vi "Read Power No Objects.vi"(8 "error in (no error)":errorcluster, 10 "VISA Resource Name":refnum<visa-resource-name>, 11 "Cluster In":T2={"Wavelength"=0.0, "AVG"=0, "Range"=0, "Backlight"=0, "Beeper"=0, "Zero"=0, "Local Lockout"=0, "ATTN"=0, "Run/Stop"=0, "Units"=0, "Averaging Time"=0.5, "Averaging"=FALSE, "Most Recent Power"=5.5, "Filter"=1} {"AVG" items=["Slow"=1, "Medium"=2, "Fast"=3]; "Range" items=["Auto", "Lowest", "2", "3", "4", "5", "6", "7", "Highest"]; "Backlight" items=["Off", "Low", "High"]; "Beeper" items=["Off", "On"]; "Zero" items=["Off", "On"]; "Local Lockout" items=["Off", "On"]; "ATTN" items=["Off", "On"]; "Run/Stop" items=["Stop", "Run"]; "Units" items=["W"=1, "dB"=2, "dBm"=3, "REL"=4]; "Filter" items=["Orange"=1, "Green"=2, "Yellow"=3]}) -> (0 "error out":errorcluster, 1 "Current Power w/ Units":string, 2 "Current Power":dbl[unit], 3 "Cluster Out":T2={"Wavelength"=0.0, "AVG"=0, "Range"=0, "Backlight"=0, "Beeper"=0, "Zero"=0, "Local Lockout"=0, "ATTN"=0, "Run/Stop"=0, "Units"=0, "Averaging Time"=0.5, "Averaging"=FALSE, "Most Recent Power"=5.5, "Filter"=1} {"AVG" items=["Slow"=1, "Medium"=2, "Fast"=3]; "Range" items=["Auto", "Lowest", "2", "3", "4", "5", "6", "7", "Highest"]; "Backlight" items=["Off", "Low", "High"]; "Beeper" items=["Off", "On"]; "Zero" items=["Off", "On"]; "Local Lockout" items=["Off", "On"]; "ATTN" items=["Off", "On"]; "Run/Stop" items=["Stop", "Run"]; "Units" items=["W"=1, "dB"=2, "dBm"=3, "REL"=4]; "Filter" items=["Orange"=1, "Green"=2, "Yellow"=3]})   [LabVIEW 2009]
doc: "Advanced Read for Power Meter.\n\nPerforms time-based Averaging based of member data. Checks for erroneous data points due to auto-ranging. Also has formatted power output."
uses:
  Newport 1830-C/Public/Filters.ctl
  Newport 1830-C/Newport 1830-C.lvlib
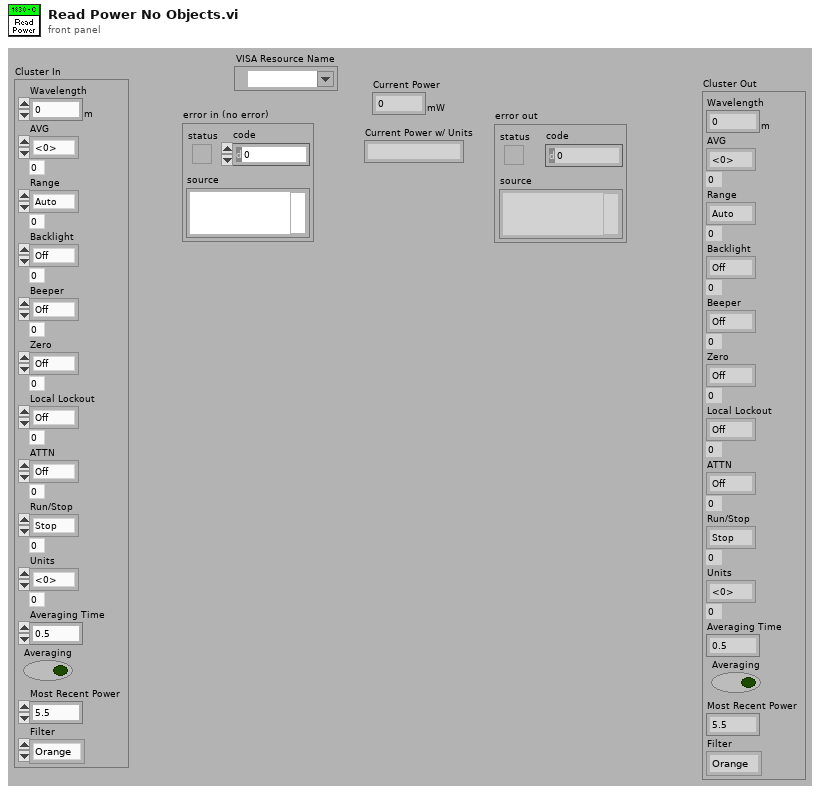
[diagram p1: front panel]
types:
  T1 = typedef "Filters.ctl" = u16
  T2 = cluster{"Wavelength":dbl[unit], "AVG":u16, "Range":u16, "Backlight":u16, "Beeper":u16, "Zero":u16, "Local Lockout":u16, "ATTN":u16, "Run/Stop":u16, "Units":u16, "Averaging Time":dbl, "Averaging":bool, "Most Recent Power":dbl, "Filter":T1}
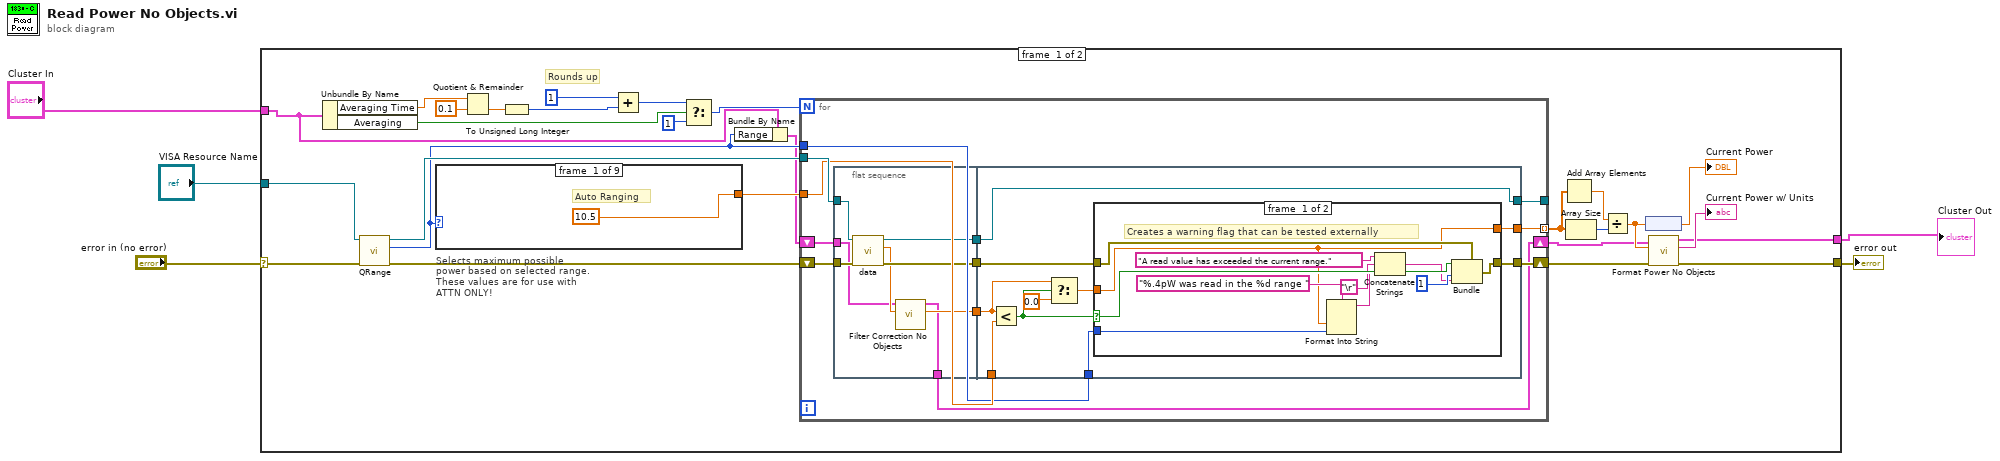
[diagram p0: block diagram]
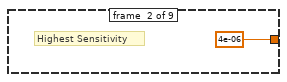
[diagram p2: hidden frame]
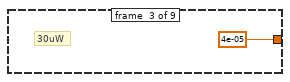
[diagram p3: hidden frame]
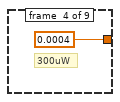
[diagram p4: hidden frame]
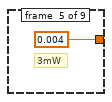
[diagram p5: hidden frame]
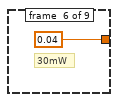
[diagram p6: hidden frame]
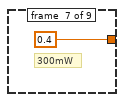
[diagram p7: hidden frame]
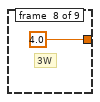
[diagram p8: hidden frame]
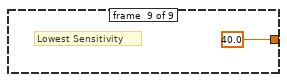
[diagram p9: hidden frame]
diagram:
  n1 = case shown="No Error" "error in (no error)" {
    selector: "error in (no error)" -> [w9 w86]
    tunnel: [w6 w86] -> w4
    tunnel: [w7 w85] -> w2
    tunnel: "VISA Resource Name" -> [w11 _]
    tunnel: "Cluster In" -> [w10 w85]
    frame #0 {
      # "Rounds up"
      n2 = Unbundle By Name(w10) -> ("Averaging Time"=w21:dbl, "Averaging"=w22:bool)
      n3 = call "QRange.vi"("error in (no error)"=w9, "VISA resource name"=w11) -> ("error out"=w16:errorcluster, "Range"=w13:u32, "VISA resource name out"=w17:refnum<visa-resource-name>)  [unwired: 7 in]
      n4 = case "Selects maximum possible\npower based on selected range.\nThese values are for use with\nATTN ONLY!" shown="4" w13 {
        tunnel: [10.5 ("y") 4e-06 ("y") 4e-05 ("y") 0.0004 ("y") 0.004 ("y") 0.04 ("y") 0.4 ("y") 4.0 ("y") 40.0 ("y")] -> w15
        frame #0 {
          # "Auto Ranging"
        }
        frame #1 {
          # "Highest Sensitivity"
        }
        frame #2 {
          # "30uW"
        }
        frame #3 {
          # "300uW"
        }
        frame #4 {
          # "3mW"
        }
        frame #5 {
          # "30mW"
        }
        frame #6 {
          # "300mW"
        }
        frame #7 {
          # "3W"
        }
        frame #8 {
          # "Lowest Sensitivity"
        }
      }
      n5 = Quotient & Remainder(x=w21, y=0.1) -> (floor(x/y)=w26:dbl)  [unwired: 1 out]
      n6 = To Unsigned Long Integer(number=w26) -> (unsigned 32bit integer=w25:u32)
      n7 = Add(x=u32 1, y=w25) -> (x+y=w29:u32)
      n8 = Select(t=w29, s=w22, f=u32 1 ("t")) -> (s? t:f=w23:u32)
      n9 = Bundle By Name(cluster=w10, "Range"=w13) -> (w12:T2)
      n10 = for {
        N: w23 -> [_]
        tunnel: w17 -> [w53]
        tunnel: [w51] -> _
        tunnel: w15 -> [w46]
        tunnel: w13 -> [w45]
        tunnel: [w44] -> w14 mode=indexing
        shift-right: [w50] -> w20
        shift-left: w16 -> [w52]
        shift-right: [w42] -> w8
        shift-left: w12 -> [w43]
        n11 = flat-sequence {
          tunnel: w53 -> [w61]
          tunnel: w52 -> [w60]
          tunnel: [w59] -> w49
          tunnel: [w58] -> w48
          tunnel: [w56] -> w47
          tunnel: w43 -> [w54]
          tunnel: [w55] -> w42
          tunnel: [w68] -> w50
          tunnel: [w71] -> w51
          tunnel: w49 -> [w71]
          tunnel: w48 -> [w69]
          tunnel: w47 -> [w66]
          tunnel: w46 -> [w67]
          tunnel: w45 -> [w64]
          tunnel: [w63] -> w44
          frame #0 {
            n12 = call "data.vi"("error in (no error)"=w60, "VISA resource name"=w61) -> ("error out"=w58:errorcluster, "Power"=w57:dbl, "VISA resource name out"=w59:refnum<visa-resource-name>)  [unwired: 7 in]
            n13 = call "Filter Correction No Objects.vi"("Read Power"=w57, "Cluster In"=w54) -> ("Corrected Power"=w56:dbl, "Cluster Out"=w55:T2)  [unwired: 8 in]
          }
          frame #1 {
            n14 = Less?(x=w66, y=w67) -> (x < y?=w62:bool)
            n15 = Select(t=w66, s=w62, f=0.0) -> (s? t:f=w65:dbl)
            n16 = case shown="False" w62 {
              selector: w62 -> [w81 _]
              tunnel: w69 -> [w82 w84]
              tunnel: [w79 w84] -> w68
              tunnel: w65 -> [w74 w83]
              tunnel: w64 -> [w75 _]
              tunnel: [w74 w83] -> w63
              frame #0 {
                # "Creates a warning flag that can be tested externally"
                n17 = Format Into String(format string="%.4pW was read in the %d range ", w74, w75) -> (resulting string=w73:string)  [unwired: 2 in, 1 out]
                n18 = Concatenate Strings("A read value has exceeded the current range." ("source"), "\r", w73) -> (w76:string)
                n19 = Bundle(cluster=w82, "status"=w81, "code"=1, "source"=w76) -> (w79:errorcluster)
              }
              frame #1 {
              }
            }
          }
        }
      }
      n20 = Add Array Elements(numeric array=w14) -> (sum=w30:dbl)
      n21 = Array Size(array=w14) -> (size(s)=w31:i32)
      n22 = Divide(x=w30, y=w31) -> (x/y=w19:dbl)
      n23 = node(w19) -> (→"Current Power":dbl[unit])
      n24 = call "Format Power No Objects.vi"("error in"=w20, "Power"=w19, "Cluster In"=w8) -> ("error out"=w6:errorcluster, "Formatted Power"=→"Current Power w/ Units":string, "Cluster Out"=w7:T2)  [unwired: 6 in]
    }
    frame #1 {
    }
  }
  "error out" <- w4
  "Cluster Out" <- w2
